vi "wd_appendCheck.vi"(8 "error in (no error)":errorcluster, 9 "DataType":T7, 10 "channel index (0)":u32, 11 "data in":T1={"TargetFile"=path "", "StreamMode"=enum."File", "Append?"=FALSE, "ChunkSize"=0, "TimeColumnMode"=enum."Empty", "TimestampFormat"="", "AbsoluteTime?"=FALSE, "FileAttribute "={"Creator"="", "Title"="", "SheetName"=""}, "Column"=[], "FileRef"=refnum, "MemoryRef"=[], "RecordInfo"=[], " ChannelPreviousInfo"=[], "ChannelFirstRecord"=[], "PredefinedFormattedValueLength"=20, "DiskTemplate"={"XMLRef"=[refnum, refnum, refnum, refnum, refnum, refnum], "ZipPath"=path "", "MetaFile"={"Ref"=refnum, "NextRow"=0, "NextPosition"=0, "Block"=[]}, "TempFolder"=path ""}}) -> (0 "error out":errorcluster, 3 "data out":T1={"TargetFile"=path "", "StreamMode"=enum."File", "Append?"=FALSE, "ChunkSize"=0, "TimeColumnMode"=enum."Empty", "TimestampFormat"="", "AbsoluteTime?"=FALSE, "FileAttribute "={"Creator"="", "Title"="", "SheetName"=""}, "Column"=[], "FileRef"=refnum, "MemoryRef"=[], "RecordInfo"=[], " ChannelPreviousInfo"=[], "ChannelFirstRecord"=[], "PredefinedFormattedValueLength"=20, "DiskTemplate"={"XMLRef"=[refnum, refnum, refnum, refnum, refnum, refnum], "ZipPath"=path "", "MetaFile"={"Ref"=refnum, "NextRow"=0, "NextPosition"=0, "Block"=[]}, "TempFolder"=path ""}})   [LabVIEW 2020, in "NI_ExcelFile.lvlib"]
uses:
  <vilib>/express/express shared/NI_ExcelFile/NI_ExcelFile.lvlib
  <vilib>/express/express shared/NI_ExcelFile/Ctrls/MainData.ctl
  <vilib>/express/express shared/NI_ExcelFile/Ctrls/StreamMode.ctl
  <vilib>/express/express shared/NI_ExcelFile/Ctrls/TimeColumnMode.ctl
  <vilib>/express/express shared/NI_ExcelFile/Ctrls/FileAttribute.ctl
  <vilib>/express/express shared/NI_ExcelFile/Ctrls/Columns.ctl
  <vilib>/express/express shared/NI_ExcelFile/Ctrls/ColumnInfo.ctl
  <vilib>/express/express shared/NI_ExcelFile/Ctrls/DataType.ctl
  <vilib>/express/express shared/NI_ExcelFile/Ctrls/wd_recordInfo.ctl
  <vilib>/express/express shared/NI_ExcelFile/Ctrls/disk_TemplateFile.ctl
  <vilib>/express/express shared/NI_ExcelFile/Ctrls/meta_file.ctl
  <vilib>/express/express shared/NI_ExcelFile/Ctrls/meta_Block.ctl
  <vilib>/express/express shared/NI_ExcelFile/Ctrls/meta_BlockType.ctl
  <vilib>/Utility/error.llb/Error Cluster From Error Code.vi
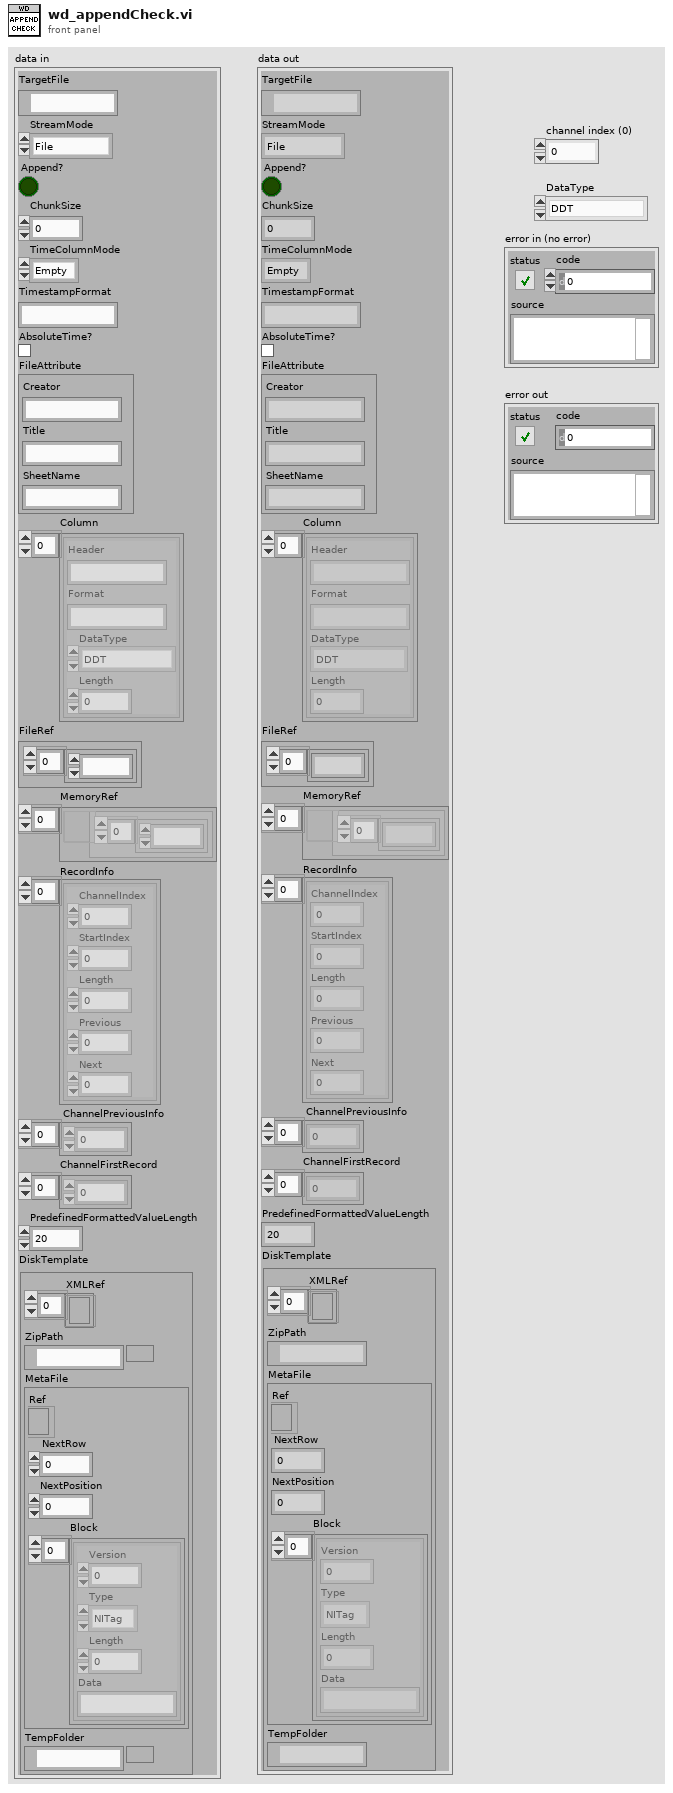
[diagram p1: front panel]
types:
  T1 = typedef "NI_ExcelFile.lvlib/MainData.ctl" = cluster{"TargetFile":path, "StreamMode":T2, "Append?":bool, "ChunkSize":u64, "TimeColumnMode":T3, "TimestampFormat":string, "AbsoluteTime?":bool, "FileAttribute ":T4, "Column":T5, "FileRef":refnum<k1>, "MemoryRef":refnum<data-value>[], "RecordInfo":T8[], " ChannelPreviousInfo":u32[], "ChannelFirstRecord":u32[], "PredefinedFormattedValueLength":i64, "DiskTemplate":T9}
  T2 = typedef "NI_ExcelFile.lvlib/StreamMode.ctl" = enum16{"File", "Memory"}
  T3 = typedef "NI_ExcelFile.lvlib/TimeColumnMode.ctl" = enum16{"Empty", "OnePerCh", "One"}
  T4 = typedef "NI_ExcelFile.lvlib/FileAttribute.ctl" = cluster{"Creator":string, "Title":string, "SheetName":string}
  T5 = typedef "NI_ExcelFile.lvlib/Columns.ctl" = T6[]
  T6 = typedef "NI_ExcelFile.lvlib/ColumnInfo.ctl" = cluster{"Header":string, "Format":string, "DataType":T7, "Length":u64}
  T7 = typedef "NI_ExcelFile.lvlib/DataType.ctl" = enum16{"DDT", "WFM", "Array of STR", "Array of DBL", "Array of I8", "Array of I16", "Array of I32", "Array of I64", "Array of SGL", "Array of U8", "Array of U16", "Array of U32", "Array of U64", "Array of Time"}
  T8 = typedef "NI_ExcelFile.lvlib/wd_recordInfo.ctl" = cluster{"ChannelIndex":u32, "StartIndex":u64, "Length":u64, "Previous":i32, "Next":i32}
  T9 = typedef "NI_ExcelFile.lvlib/disk_TemplateFile.ctl" = cluster{"XMLRef":refnum<file>[], "ZipPath":path, "MetaFile":T10, "TempFolder":path}
  T10 = typedef "NI_ExcelFile.lvlib/meta_file.ctl" = cluster{"Ref":refnum<file>, "NextRow":i32, "NextPosition":i64, "Block":T11[]}
  T11 = typedef "NI_ExcelFile.lvlib/meta_Block.ctl" = cluster{"Version":u16, "Type":T12, "Length":i32, "Data":string}
  T12 = typedef "NI_ExcelFile.lvlib/meta_BlockType.ctl" = enum16{"NITag", "File", "Column"}
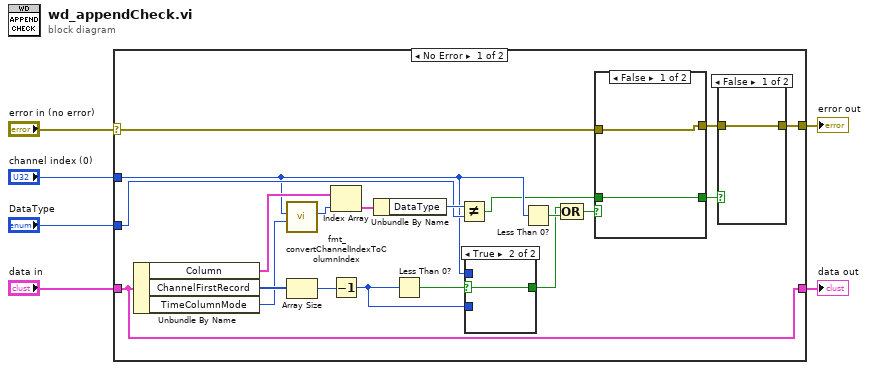
[diagram p0: block diagram]
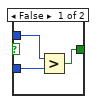
[diagram p2: hidden frame]
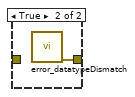
[diagram p3: hidden frame]
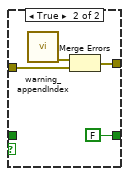
[diagram p4: hidden frame]
diagram:
  n1 = case shown="No Error" "error in (no error)" {
    selector: "error in (no error)" -> [w14 w40]
    tunnel: "data in" -> [w15 w39]
    tunnel: "channel index (0)" -> [w11 _]
    tunnel: "DataType" -> [w20 _]
    tunnel: [w15 w39] -> w2
    tunnel: [w18 w40] -> w1
    frame No Error {
      n2 = Unbundle By Name(w15) -> ("Column"=w24:T5, "ChannelFirstRecord"=w23:u32[], "TimeColumnMode"=w17:T3)
      n3 = call <vilib>:"fmt_convertChannelIndexToColumnIndex.vi"("TimeColumnMode"=w17, "channel index"=w11) -> ("data column index"=w16:i32)  [unwired: 8 in, 1 out]
      n4 = Array Size(array=w23) -> (size(s)=w21:i32)
      n5 = Index Array(array=w24, index=w16) -> (element=w25:T6)
      n6 = Decrement(x=w21) -> (x-1=w10:i32)
      n7 = Unbundle By Name(w25) -> ("DataType"=w26:T7)
      n8 = Less Than 0?(x=w10) -> (x < 0?=w13:bool)
      n9 = Not Equal?(x=w26, y=w20) -> (x != y?=w9:bool)
      n10 = case shown="True" w13 {
        selector: w13 -> [_ w30]
        tunnel: [w27 w30] -> w12
        tunnel: w11 -> [w29 _]
        tunnel: w10 -> [w28 _]
        frame False {
          n11 = Greater?(x=w29, y=w28) -> (0:w27:bool)
        }
        frame True {
        }
      }
      n12 = Less Than 0?(x=w11) -> (x < 0?=w22:bool)
      n13 = Compound Arithmetic op=OR(w12, w22) -> (w19:bool)
      n14 = case shown="False" w19 {
        tunnel: w14 -> [w34 w38]
        tunnel: [w34 w37] -> w7
        tunnel: w9 -> [w33 _]
        tunnel: [w33 FALSE] -> w8
        frame False {
        }
        frame True {
          n15 = call <vilib>:"warning_appendIndex.vi"() -> ("error out"=w36:errorcluster)  [unwired: 11 in]
          n16 = Merge Errors(w36, w38) -> (w37:errorcluster)
        }
      }
      n17 = case shown="False" w8 {
        tunnel: [w31 w32] -> w18
        tunnel: w7 -> [w31 _]
        frame False {
        }
        frame True {
          n18 = call <vilib>:"error_datatypeDismatch.vi"() -> ("error out"=w32:errorcluster)  [unwired: 11 in]
        }
      }
    }
    frame Error {
    }
  }
  "error out" <- w1
  "data out" <- w2
